vi "SIFT align.vi"(6 "post image file":string="post.png", 7 "pre image file":string="pre.png", 8 "Inverse PNG":bool=TRUE, 9 "Affine":bool, 10 "smoothing radius":u16=2, 11 "working directory":path=path "D:/3D FIB-SEM Files") -> (0 "Delta image":dbl format="%#_3g", 1 "failed":bool, 2 "Delta Y":dbl format="%#_3g", 3 "Delta X":dbl format="%#_3g", 4 "align post image":u8[][](array[numeric]), 5 "pre image":u8[][](array[numeric]))   [LabVIEW 2018]
panel:
  out "Translation array":dbl[](array[numeric])
  out "Affine array":dbl[](array[numeric])
  out "SIFT.txt":string
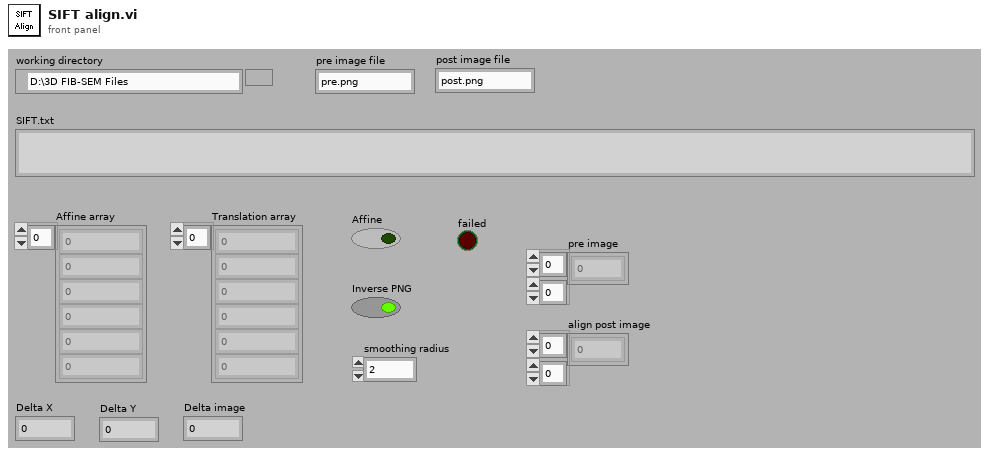
[diagram p1: front panel]
types:
  T1 = enum16{"open", "replace", "create", "open or create", "replace or create", "replace or create with confirmation"}
  T2 = typedef "imagedata.ctl" = cluster{"image type":i32, "image depth":i32, "image":u8[], "mask":u8[], "colors":u32[], "Rectangle":cluster{"left":i16, "top":i16, "right":i16, "bottom":i16}}
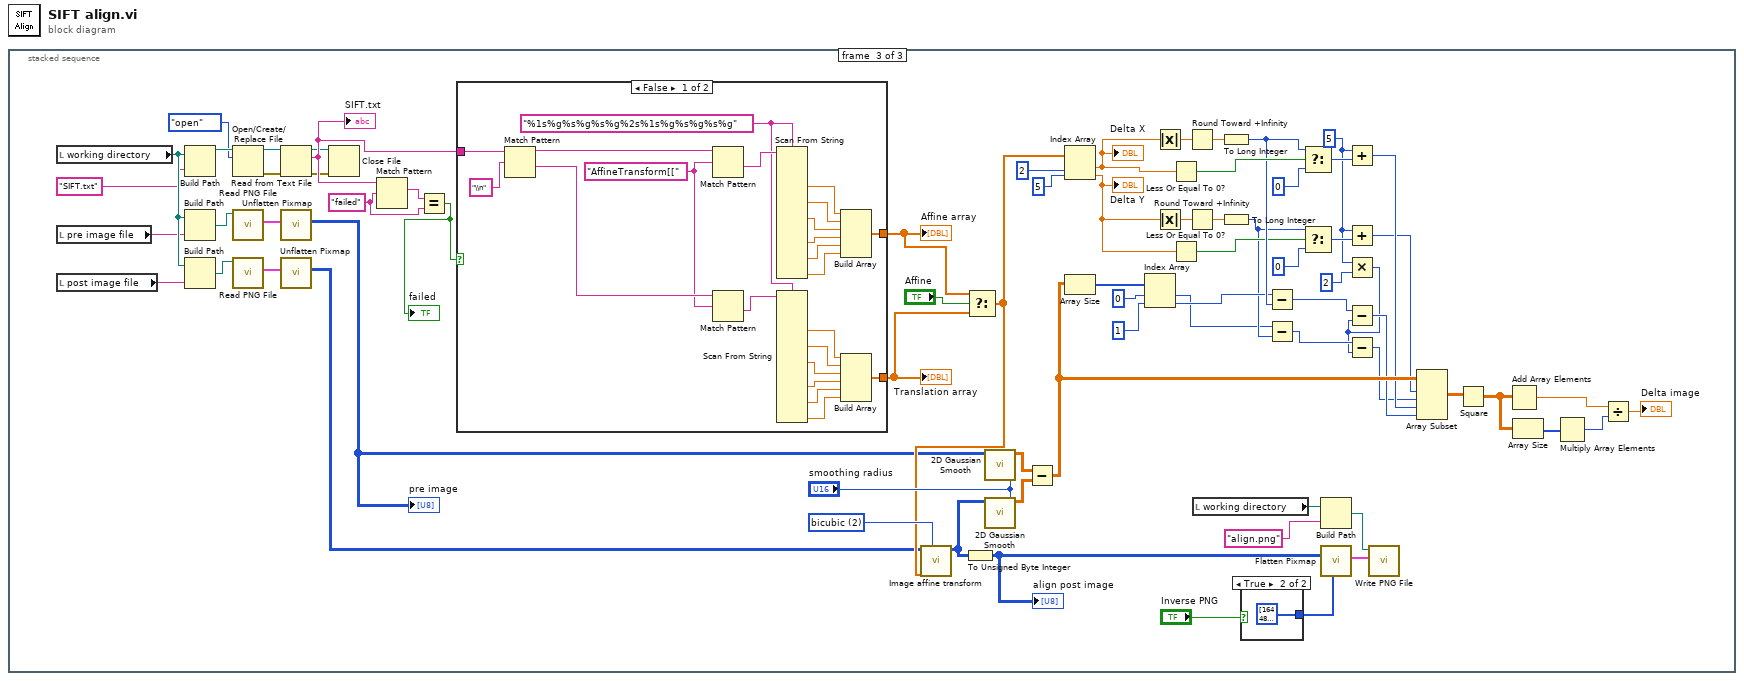
[diagram p0: block diagram]
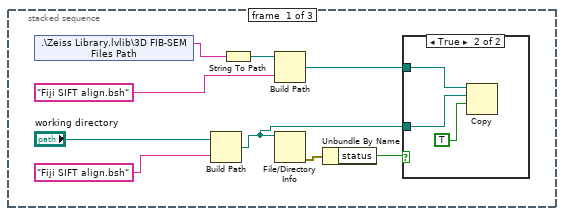
[diagram p2: hidden frame]
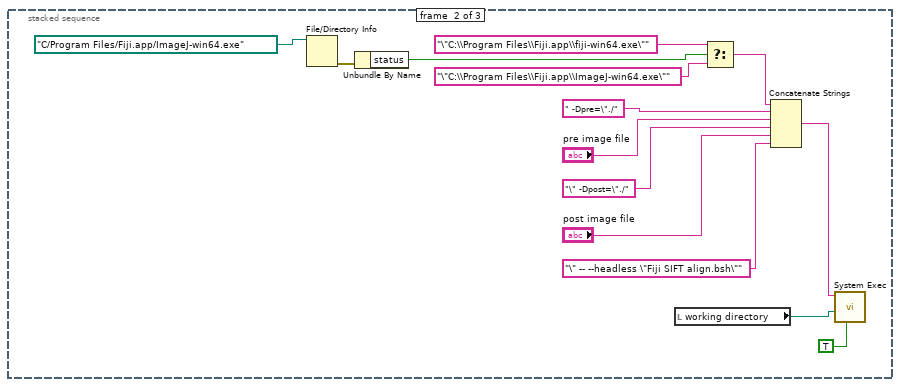
[diagram p4: hidden frame]
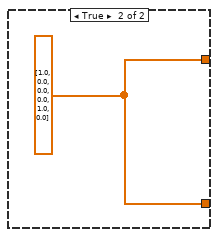
[diagram p5: hidden frame]
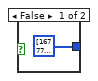
[diagram p6: hidden frame]
diagram:
  n1 = stacked-sequence {
    frame #0 {
      n2 = shared-variable ".\\Zeiss Library.lvlib\\3D FIB-SEM Files Path"() -> (w2:string)  [unwired: 1 in, 1 out]
      n3 = Build Path(base path="working directory", name or relative path="Fiji SIFT align.bsh") -> (appended path=w5:path)
      n4 = String To Path(string=w2) -> (path=w1:path)
      n5 = Build Path(base path=w1, name or relative path="Fiji SIFT align.bsh") -> (appended path=w3:path)
      n6 = File/Directory Info(path=w5) -> (error out=w7:errorcluster)  [unwired: 1 in, 6 out]
      n7 = Unbundle By Name(w7) -> ("status"=w6:bool)
      n8 = case shown="True" w6 {
        tunnel: w5 -> [_ w11]
        tunnel: w3 -> [_ w10]
        frame False {
        }
        frame True {
          n9 = Copy(9:TRUE ("run minimized? (F)"), 10:w11, 11:w10) -> ()  [unwired: 2 in, 3 out]
        }
      }
    }
    frame #1 {
      n10 = File/Directory Info(path=path "C:/Program Files/Fiji.app/ImageJ-win64.exe") -> (error out=w24:errorcluster)  [unwired: 1 in, 6 out]
      n11 = Unbundle By Name(w24) -> ("status"=w22:bool)
      n12 = local read "working directory"() -> (w13:path)
      n13 = Select(t="\"C:\\Program Files\\Fiji.app\\fiji-win64.exe\"" ("command line"), s=w22, f="\"C:\\Program Files\\Fiji.app\\ImageJ-win64.exe\"" ("command line")) -> (s? t:f=w20:string)
      n14 = Concatenate Strings(w20, " -Dpre=\"./" ("string"), "pre image file", "\" -Dpost=\"./" ("string"), "post image file", "\" -- --headless \"Fiji SIFT align.bsh\"" ("string")) -> (w19:string)
      n15 = call <vilib>:"System Exec.vi"("run minimized? (F)"=TRUE, "working directory"=w13, "command line"=w19) -> ()  [unwired: 5 in, 4 out]
    }
    frame #2 {
      w33 = 5 ("x")
      w64 = "failed" ("regular expression")
      w86 = 2 items=["nearest", "bilinear", "bicubic", "bicubic spline"] ("method")
      n16 = local read "working directory"() -> (w92:path)
      n17 = local read "pre image file"() -> (w29:string)
      n18 = local read "post image file"() -> (w28:string)
      n19 = Build Path(base path=w92, name or relative path="SIFT.txt") -> (appended path=w99:path)
      n20 = Build Path(base path=w92, name or relative path=w29) -> (appended path=w91:path)
      n21 = Build Path(base path=w92, name or relative path=w28) -> (appended path=w93:path)
      n22 = Open/Create/Replace File(file path (use dialog)=w99, operation (0:open)=T1."open") -> (refnum out=w97:refnum<file>, error out=w96:errorcluster)  [unwired: 4 in, 1 out]
      n23 = call <vilib>:"Read PNG File.vi"("path to PNG file"=w91) -> ("image data"=w95:T2)  [unwired: 8 in, 2 out]
      n24 = call <vilib>:"Read PNG File.vi"("path to PNG file"=w93) -> ("image data"=w94:T2)  [unwired: 8 in, 2 out]
      n25 = Read from Text File(file (use dialog)=w97, error in=w96) -> (refnum out=w60:refnum<file>, text=w66:string, error out=w61:errorcluster)  [unwired: 2 in, 1 out]
      "SIFT.txt" <- w66
      n26 = call <vilib>:"Unflatten Pixmap.vi"("image data"=w95) -> ("8-bit pixmap"=w27:u8[][])  [unwired: 4 in, 6 out]
      "pre image" <- w27
      n27 = call <vilib>:"Unflatten Pixmap.vi"("image data"=w94) -> ("8-bit pixmap"=w62:u8[][])  [unwired: 4 in, 6 out]
      n28 = Close File(refnum=w60, error in=w61) -> ()  [unwired: 2 out]
      n29 = Match Pattern(string=w66, regular expression=w64) -> (match substring=w65:string)  [unwired: 1 in, 3 out]
      n30 = Equal?(x=w65, y=w64) -> (x = y?=w63:bool)
      "failed" <- w63
      n31 = case shown="False" w63 {
        tunnel: [w102 w122] -> w74
        tunnel: [w101 w122] -> w73
        tunnel: w66 -> [w100 _]
        frame False {
          w103 = "%1s%g%s%g%s%g%2s%1s%g%s%g%s%g" ("format string")
          w104 = "AffineTransform[[" ("regular expression")
          n32 = Match Pattern(string=w100, regular expression="\\n") -> (before substring=w120:string, after substring=w105:string)  [unwired: 1 in, 2 out]
          n33 = Match Pattern(string=w120, regular expression=w104) -> (after substring=w119:string)  [unwired: 1 in, 3 out]
          n34 = Match Pattern(string=w105, regular expression=w104) -> (after substring=w106:string)  [unwired: 1 in, 3 out]
          n35 = Scan From String(format string=w103, input string=w119) -> (output 2=w118:dbl, output 4=w117:dbl, output 6=w116:dbl, output 9=w115:dbl, output 11=w114:dbl, output 13=w113:dbl)  [unwired: 22 in, 3 out]
          n36 = Scan From String(format string=w103, input string=w106) -> (output 2=w107:dbl, output 4=w108:dbl, output 6=w109:dbl, output 9=w110:dbl, output 11=w111:dbl, output 13=w112:dbl)  [unwired: 22 in, 3 out]
          n37 = Build Array(w118, w117, w116, w115, w114, w113) -> (w102:dbl[])
          n38 = Build Array(w107, w108, w109, w110, w111, w112) -> (w101:dbl[])
        }
        frame True {
          w122 = dbl[] [1.0, 0.0, 0.0, 0.0, 1.0, 0.0]
        }
      }
      "Affine array" <- w74
      "Translation array" <- w73
      n39 = Select(t=w74, s="Affine", f=w73) -> (s? t:f=w71:dbl[])
      n40 = call "Image affine transform.vi"("method"=w86, "Affine array"=w71, "Input image"=w62) -> ("Output image"=w79:i16[][])  [unwired: 8 in]
      n41 = To Unsigned Byte Integer(number=w79) -> (unsigned 8bit integer=w81:u8[][])
      "align post image" <- w81
      n42 = call "2D Gaussian Smooth.vi"("radius"="smoothing radius", "Input"=w27) -> ("Output"=w77:dbl[][])  [unwired: 8 in, 1 out]
      n43 = call "2D Gaussian Smooth.vi"("radius"="smoothing radius", "Input"=w79) -> ("Output"=w78:dbl[][])  [unwired: 8 in, 1 out]
      n44 = Subtract(x=w77, y=w78) -> (x-y=w59:dbl[][])
      n45 = Index Array(array=w71, index #1=2 ("index"), index #2=5 ("index")) -> (element #1=w55:dbl, element #2=w44:dbl)
      "Delta X" <- w55
      "Delta Y" <- w44
      n46 = Array Size(array=w59) -> (size(s)=w58:i32[])
      n47 = Index Array(array=w58, index #1=0 ("index"), index #2=1 ("index")) -> (element #1=w42:i32, element #2=w49:i32)
      n48 = Absolute Value(x=w55) -> (abs(x)=w54:dbl)
      n49 = Absolute Value(x=w44) -> (abs(x)=w45:dbl)
      n50 = Less Or Equal To 0?(x=w55) -> (x <= 0?=w52:bool)
      n51 = Less Or Equal To 0?(x=w44) -> (x <= 0?=w47:bool)
      n52 = Round Toward +Infinity(x=w54) -> (ceil(x): smallest int >= x=w53:dbl)
      n53 = Round Toward +Infinity(x=w45) -> (ceil(x): smallest int >= x=w46:dbl)
      n54 = local read "working directory"() -> (w88:path)
      n55 = To Long Integer(number=w53) -> (32bit integer=w50:i32)
      n56 = To Long Integer(number=w46) -> (32bit integer=w43:i32)
      n57 = case shown="True" "Inverse PNG" {
        tunnel: [u32[] [16777222, 65793, 131586, 197379, 263172, 328965, 394758, 460551, 526344, 592137, 657930, 723723, 789516, 855309, 921102, 986895, 1052688, 1118481, 1184274, 1250067, 1315860, 1381653, 1447446, 1513239, 1579032, 1644825, 1710618, 1776411, 1842204, 1907997, 1973790, 2039583, 2105376, 2171169, 2236962, 2302755, 2368548, 2434341, 2500134, 2565927, 2631720, 2697513, 2763306, 2829099, 2894892, 2960685, 3026478, 3092271, 3158064, 3223857, 3289650, 3355443, 3421236, 3487029, 3552822, 3618615, 3684408, 3750201, 3815994, 3881787, 3947580, 4013373, 4079166, 4144959, 4210752, 4276545, 4342338, 4408131, 4473924, 4539717, 4605510, 4671303, 4737096, 4802889, 4868682, 4934475, 5000268, 5066061, 5131854, 5197647, 5263440, 5329233, 5395026, 5460819, 5526612, 5592405, 5658198, 5723991, 5789784, 5855577, 5921370, 5987163, 6052956, 6118749, 6184542, 6250335, 6316128, 6381921, 6447714, 6513507, 6579300, 6645093, 6710886, 6776679, 6842472, 6908265, 6974058, 7039851, 7105644, 7171437, 7237230, 7303023, 7368816, 7434609, 7500402, 7566195, 7631988, 7697781, 7763574, 7829367, 7895160, 7960953, 8026746, 8092539, 8158332, 8224125, 8289918, 8355711, 8421504, 8487297, 8553090, 8618883, 8684676, 8750469, 8816262, 8882055, 8947848, 9013641, 9079434, 9145227, 9211020, 9276813, 9342606, 9408399, 9474192, 9539985, 9605778, 9671571, 9737364, 9803157, 9868950, 9934743, 10000536, 10066329, 10132122, 10197915, 10263708, 10329501, 10395294, 10461087, 10526880, 10592673, 10658466, 10724259, 10790052, 10855845, 10921638, 10987431, 11053224, 11119017, 11184810, 11250603, 11316396, 11382189, 11447982, 11513775, 11579568, 11645361, 11711154, 11776947, 11842740, 11908533, 11974326, 12040119, 12105912, 12171705, 12237498, 12303291, 12369084, 12434877, 12500670, 12566463, 12632256, 12698049, 12763842, 12829635, 12895428, 12961221, 13027014, 13092807, 13158600, 13224393, 13290186, 13355979, 13421772, 13487565, 13553358, 13619151, 13684944, 13750737, 13816530, 13882323, 13948116, 14013909, 14079702, 14145495, 14211288, 14277081, 14342874, 14408667, 14474460, 14540253, 14606046, 14671839, 14737632, 14803425, 14869218, 14935011, 15000804, 15066597, 15132390, 15198183, 15263976, 15329769, 15395562, 15461355, 15527148, 15592941, 15658734, 15724527, 15790320, 15856113, 15921906, 15987699, 16053492, 16119285, 16185078, 16250871, 16316664, 16382457, 16448250, 16514043, 16579836, 16645629, 16711422, 16448250] ("256 gray scale") u32[] [16448250, 16711422, 16645629, 16579836, 16514043, 16448250, 16382457, 16316664, 16250871, 16185078, 16119285, 16053492, 15987699, 15921906, 15856113, 15790320, 15724527, 15658734, 15592941, 15527148, 15461355, 15395562, 15329769, 15263976, 15198183, 15132390, 15066597, 15000804, 14935011, 14869218, 14803425, 14737632, 14671839, 14606046, 14540253, 14474460, 14408667, 14342874, 14277081, 14211288, 14145495, 14079702, 14013909, 13948116, 13882323, 13816530, 13750737, 13684944, 13619151, 13553358, 13487565, 13421772, 13355979, 13290186, 13224393, 13158600, 13092807, 13027014, 12961221, 12895428, 12829635, 12763842, 12698049, 12632256, 12566463, 12500670, 12434877, 12369084, 12303291, 12237498, 12171705, 12105912, 12040119, 11974326, 11908533, 11842740, 11776947, 11711154, 11645361, 11579568, 11513775, 11447982, 11382189, 11316396, 11250603, 11184810, 11119017, 11053224, 10987431, 10921638, 10855845, 10790052, 10724259, 10658466, 10592673, 10526880, 10461087, 10395294, 10329501, 10263708, 10197915, 10132122, 10066329, 10000536, 9934743, 9868950, 9803157, 9737364, 9671571, 9605778, 9539985, 9474192, 9408399, 9342606, 9276813, 9211020, 9145227, 9079434, 9013641, 8947848, 8882055, 8816262, 8750469, 8684676, 8618883, 8553090, 8487297, 8421504, 8355711, 8289918, 8224125, 8158332, 8092539, 8026746, 7960953, 7895160, 7829367, 7763574, 7697781, 7631988, 7566195, 7500402, 7434609, 7368816, 7303023, 7237230, 7171437, 7105644, 7039851, 6974058, 6908265, 6842472, 6776679, 6710886, 6645093, 6579300, 6513507, 6447714, 6381921, 6316128, 6250335, 6184542, 6118749, 6052956, 5987163, 5921370, 5855577, 5789784, 5723991, 5658198, 5592405, 5526612, 5460819, 5395026, 5329233, 5263440, 5197647, 5131854, 5066061, 5000268, 4934475, 4868682, 4802889, 4737096, 4671303, 4605510, 4539717, 4473924, 4408131, 4342338, 4276545, 4210752, 4144959, 4079166, 4013373, 3947580, 3881787, 3815994, 3750201, 3684408, 3618615, 3552822, 3487029, 3421236, 3355443, 3289650, 3223857, 3158064, 3092271, 3026478, 2960685, 2894892, 2829099, 2763306, 2697513, 2631720, 2565927, 2500134, 2434341, 2368548, 2302755, 2236962, 2171169, 2105376, 2039583, 1973790, 1907997, 1842204, 1776411, 1710618, 1644825, 1579032, 1513239, 1447446, 1381653, 1315860, 1250067, 1184274, 1118481, 1052688, 986895, 921102, 855309, 789516, 723723, 657930, 592137, 526344, 460551, 394758, 328965, 263172, 197379, 131586, 65793, 16777222] ("256 gray scale inverse")] -> w68
        frame False {
        }
        frame True {
        }
      }
      n58 = Subtract(x=w49, y=w50) -> (x-y=w37:i32)
      n59 = Subtract(x=w42, y=w43) -> (x-y=w35:i32)
      n60 = Select(t=w50, s=w52, f=0 ("element")) -> (s? t:f=w41:i32)
      n61 = Select(t=w43, s=w47, f=0 ("element")) -> (s? t:f=w38:i32)
      n62 = Build Path(base path=w88, name or relative path="align.png") -> (appended path=w87:path)
      n63 = call <vilib>:"Flatten Pixmap.vi"("colors"=w68, "8-bit pixmap"=w81) -> ("image data"=w90:T2)  [unwired: 4 in, 5 out]
      n64 = Add(x=w33, y=w41) -> (x+y=w40:i32)
      n65 = Add(x=w33, y=w38) -> (x+y=w39:i32)
      n66 = Multiply(x=w33, y=2) -> (x*y=w31:i32)
      n67 = Subtract(x=w37, y=w31) -> (x-y=w36:i32)
      n68 = Subtract(x=w35, y=w31) -> (x-y=w34:i32)
      n69 = call <vilib>:"Write PNG File.vi"("image data"=w90, "path to PNG file"=w87) -> ()  [unwired: 8 in, 2 out]
      n70 = Array Subset(array=w59, index (row)=w39, length (row)=w34, index (col)=w40, length (col)=w36) -> (w85:dbl[][])
      n71 = Square(x=w85) -> (x^2=w80:dbl[][])
      n72 = Add Array Elements(numeric array=w80) -> (sum=w83:dbl)
      n73 = Array Size(array=w80) -> (size(s)=w84:i32[])
      n74 = Multiply Array Elements(1:w84) -> (0:w82:i32)
      n75 = Divide(x=w83, y=w82) -> (x/y=→"Delta image":dbl)
    }
  }
